vi "apply_zoom_factor.vi"(8 "error in (no error)":errorcluster, 11 "TrajectoryMH100122AODRAPS in":refnum<class "TrajectoryMH100122AODRAPS.lvclass">) -> (0 "error out":errorcluster, 3 "TrajectoryMH100122AODRAPS out":refnum<class "TrajectoryMH100122AODRAPS.lvclass">)   [LabVIEW 2010, in "TrajectoryMH100122AODRAPS.lvclass"]
uses:
  TrajectoryMH100122AODRAPS.lvclass
  TrajectoryMH100122AODRAPS.lvclass/TrajectoryMH100122AODRAPS.ctl
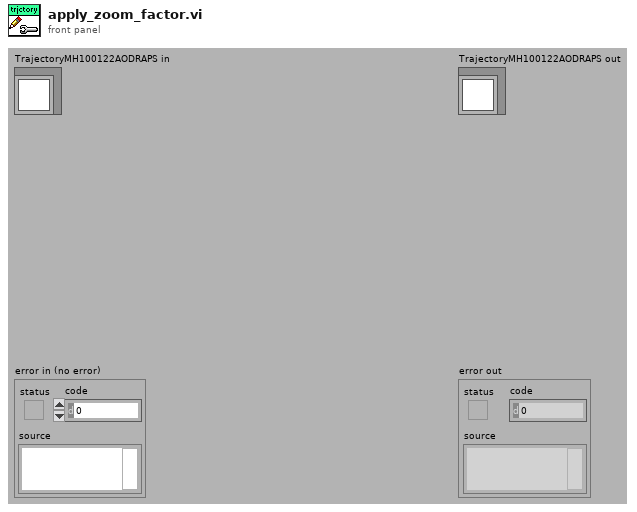
[diagram p1: front panel]
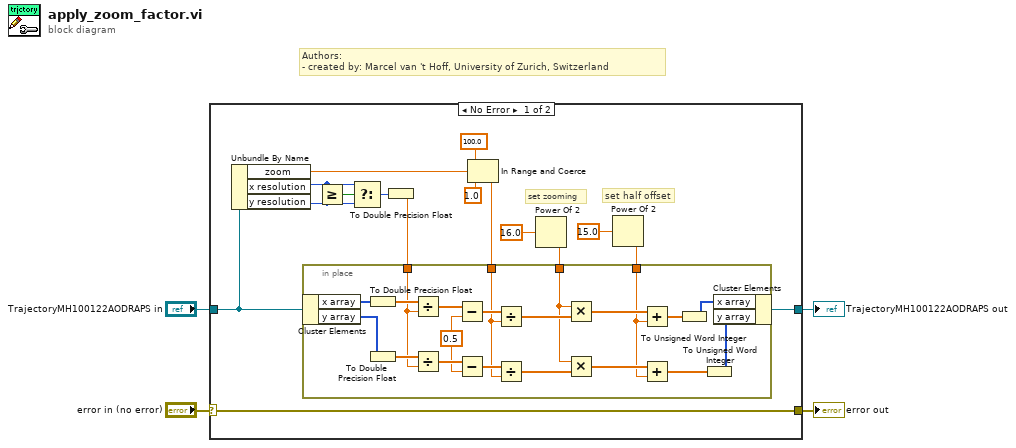
[diagram p0: block diagram]
diagram:
  # "Authors: \n- created by: Marcel van 't Hoff, University of Zurich, Switzerland"
  n1 = case shown="No Error" "error in (no error)" {
    selector: "error in (no error)" -> [w20 w43]
    tunnel: [w20 w43] -> w3
    tunnel: [w5 w42] -> w1
    tunnel: "TrajectoryMH100122AODRAPS in" -> [w6 w42]
    frame No Error {
      # "set half offset"
      # "set zooming"
      n2 = Unbundle By Name(w6) -> ("zoom"=w11:dbl, "x resolution"=w17:u32, "y resolution"=w16:u32)
      n3 = Greater Or Equal?(x=w17, y=w16) -> (x >= y?=w18:bool)
      n4 = Select(t=w17, s=w18, f=w16) -> (s? t:f=w19:u32)
      n5 = To Double Precision Float(number=w19) -> (double precision float=w15:dbl)
      n6 = In Range and Coerce(upper limit=100.0, x=w11, lower limit=1.0) -> (coerced(x)=w12:dbl)  [unwired: 1 out]
      n7 = Power Of 2(x=16.0) -> (2^x=w9:dbl)
      n8 = Power Of 2(x=15.0) -> (2^x=w7:dbl)
      n9 = in-place {
        in-place-border: w15 -> [w37]
        in-place-border: w12 -> [w31]
        in-place-border: w9 -> [w28]
        in-place-border: w7 -> [w25]
        w34 = 0.5 ("y")
        n10 = in-place-cluster #1(w6) -> ("x array"=w40:u16[], "y array"=w41:u16[])
        n11 = To Double Precision Float(number=w40) -> (double precision float=w39:dbl[])
        n12 = To Double Precision Float(number=w41) -> (double precision float=w38:dbl[])
        n13 = Divide(x=w39, y=w37) -> (x/y=w36:dbl[])
        n14 = Divide(x=w38, y=w37) -> (x/y=w35:dbl[])
        n15 = Subtract(x=w36, y=w34) -> (x-y=w33:dbl[])
        n16 = Subtract(x=w35, y=w34) -> (x-y=w32:dbl[])
        n17 = Divide(x=w33, y=w31) -> (x/y=w30:dbl[])
        n18 = Divide(x=w32, y=w31) -> (x/y=w29:dbl[])
        n19 = Multiply(x=w28, y=w30) -> (x*y=w27:dbl[])
        n20 = Multiply(x=w28, y=w29) -> (x*y=w26:dbl[])
        n21 = Add(x=w27, y=w25) -> (x+y=w24:dbl[])
        n22 = Add(x=w26, y=w25) -> (x+y=w22:dbl[])
        n23 = To Unsigned Word Integer(number=w24) -> (unsigned 16bit integer=w23:u16[])
        n24 = To Unsigned Word Integer(number=w22) -> (unsigned 16bit integer=w21:u16[])
        n25 = in-place-cluster #1("x array"=w23, "y array"=w21) -> (w5:refnum<class "TrajectoryMH100122AODRAPS.lvclass">)
      }
    }
    frame Error {
    }
  }
  "error out" <- w3
  "TrajectoryMH100122AODRAPS out" <- w1
